vi "Create Websockets Connection.vi"(5 "WSConnection in":refnum<class "WebsocketsConnection.lvclass">, 8 "error in (no error)":errorcluster, 11 "WebSocket":refnum<class "WebSocket.lvclass">) -> (0 "error out":errorcluster, 3 "WSConnection":refnum<class "WebsocketsConnection.lvclass">)   [LabVIEW 2013, in "MQTT_Websockets.lvlib" / "WebsocketsConnection.lvclass"]
uses:
  WebsocketsConnection.lvclass
  <vilib>/MediaMongrels Ltd/WebSockets/WebSockets/WebSocket/WebSocket.lvclass
  WebsocketsConnection.lvclass/WebsocketsConnection.ctl
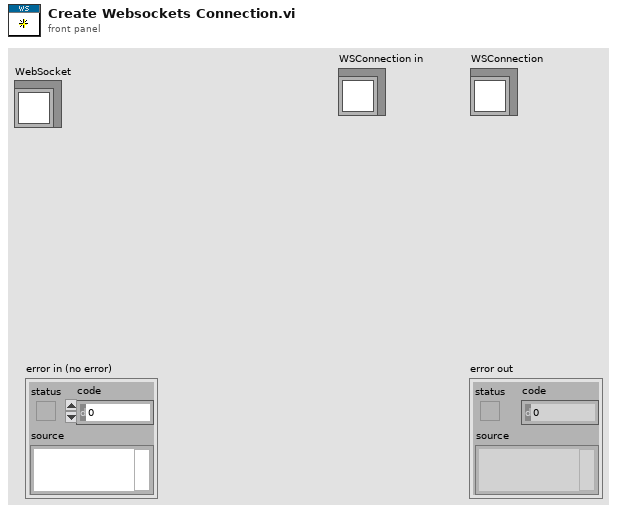
[diagram p1: front panel]
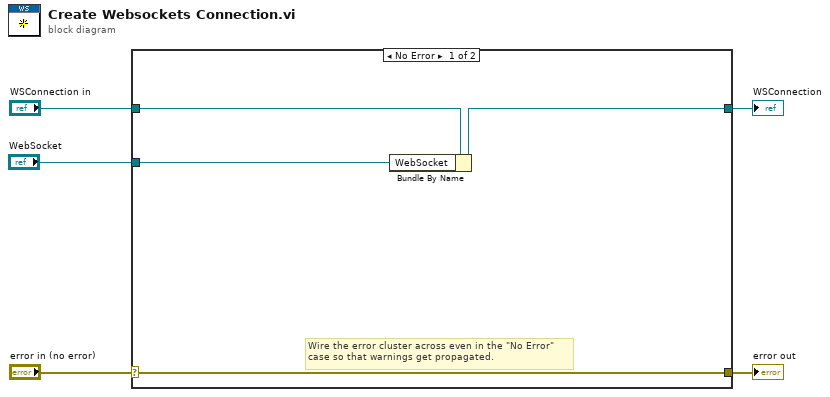
[diagram p0: block diagram]
diagram:
  n1 = case shown="No Error" "error in (no error)" {
    selector: "error in (no error)" -> [w8 w11]
    tunnel: [w8 w11] -> w4
    tunnel: [w7 w10] -> w2
    tunnel: "WSConnection in" -> [w9 w10]
    tunnel: "WebSocket" -> [w6 _]
    frame No Error {
      # "Wire the error cluster across even in the \"No Error\"\ncase so that warnings get propagated."
      n2 = Bundle By Name(cluster=w9, "WebSocket"=w6) -> (w7:refnum<class "WebsocketsConnection.lvclass">)
    }
    frame Error {
    }
  }
  "error out" <- w4
  "WSConnection" <- w2
